vi "MSEditor_SaveScriptFile.vi"(8 "error in (no error)":errorcluster, 10 "Script":string, 11 "Path in":path) -> (0 "error out":errorcluster, 3 "path out":path)   [LabVIEW 2018]
uses:
  <userlib>/_OpenG.lib/file/file.llb/Valid Path - Traditional__ogtk.vi
  <userlib>/_OpenG.lib/file/file.llb/File Exists - Scalar__ogtk.vi
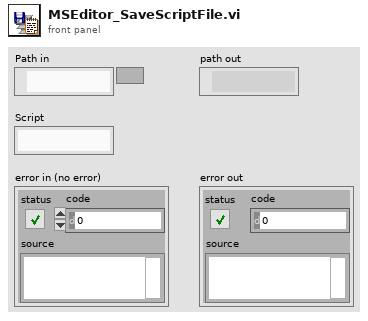
[diagram p1: front panel]
types:
  T1 = enum16{"open", "replace", "create", "open or create", "replace or create", "replace or create with confirmation"}
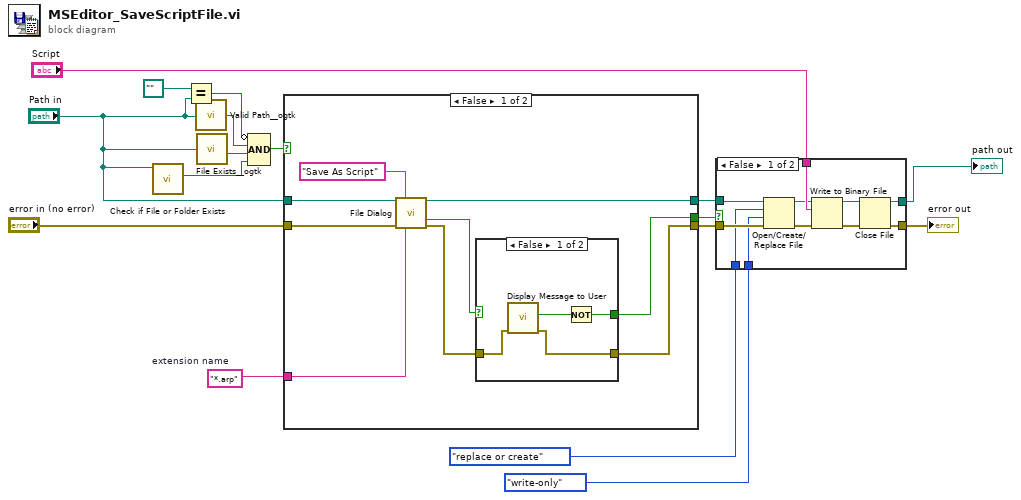
[diagram p0: block diagram]
diagram:
  w17 = "*.arp"  # extension name
  n1 = call <vilib>:"Check if File or Folder Exists.vi"("path"="Path in") -> ("file or folder exists?"=w5:bool)  [unwired: 8 in, 2 out]
  n2 = Equal?(x=path "", y="Path in") -> (x = y?=w2:bool)
  n3 = call-poly <userlib>:"Valid Path__ogtk.vi"("path"="Path in") -> ("valid"=w16:bool)
  n4 = call-poly <userlib>:"File Exists__ogtk.vi"("file path"="Path in") -> ("exists"=w13:bool)  [unwired: 6 in, 1 out]
  n5 = Compound Arithmetic op=AND(invert w2, w16, w13, w5) -> (w15:bool)
  n6 = case shown="False" w15 {
    tunnel: [w26 w34] -> w9
    tunnel: w17 -> [w25 _]
    tunnel: [w21 w33] -> w10
    tunnel: "Path in" -> [w24 w34]
    tunnel: "error in (no error)" -> [w23 w33]
    tunnel: [w19 _] -> w1
    frame False {
      n7 = call "File Dialog"("start path"=w24, "prompt"="Save As Script", "error in"=w23, "pattern (all files)"=w25) -> ("selected path"=w26:path, "cancelled"=w20:bool, "error out"=w22:errorcluster)  [unwired: 8 in, 1 out]
      n8 = case shown="False" w20 {
        selector: w20 -> [_ w32]
        tunnel: w22 -> [w30 w31]
        tunnel: [w29 w31] -> w21
        tunnel: [w27 w32] -> w19
        frame False {
          n9 = call "Display Message to User"("error in (no error)"=w30) -> ("error out"=w29:errorcluster, "OK"=w28:bool)  [unwired: 9 in]
          n10 = Not(x=w28) -> (.not. x?=w27:bool)
        }
        frame True {
        }
      }
    }
    frame True {
    }
  }
  n11 = case shown="False" w1 {
    tunnel: [w45 w47] -> w12
    tunnel: [w44 w46] -> w11
    tunnel: w10 -> [w43 w46]
    tunnel: w9 -> [w42 w47]
    tunnel: "Script" -> [w39 _]
    tunnel: enum16{"read/write", "read-only", "write-only"}."write-only" ("access (0:read/write)") -> [w36 _]
    tunnel: T1."replace or create" ("operation (0:open)") -> [w35 _]
    frame False {
      n12 = Open/Create/Replace File(file path (use dialog)=w42, error in=w43, operation (0:open)=w35, access (0:read/write)=w36) -> (refnum out=w37:refnum<file>, error out=w38:errorcluster)  [unwired: 2 in, 1 out]
      n13 = Write to Binary File(file (use dialog)=w37, data=w39, error in=w38) -> (refnum out=w40:refnum<file>, error out=w41:errorcluster)  [unwired: 3 in, 1 out]
      n14 = Close File(refnum=w40, error in=w41) -> (path=w45:path, error out=w44:errorcluster)
    }
    frame True {
    }
  }
  "path out" <- w12
  "error out" <- w11
